vi "dectector.vi"() -> ()   [LabVIEW 2014]
uses:
  <vilib>/Analysis/2dsp.llb/1D Cross Correlation (DBL).vi
  <vilib>/Analysis/NI_AALBase.lvlib
  <vilib>/Analysis/NI_AALPro.lvlib
panel:
  out "size(s)":i32
  out "sinewave":dbl[](graph)
  out "Autocorrelacion":dynamicdata(graph)
  in  "Muestras":i32=128
  in  "Amplitud":dbl=1.0 format="%#_13g"
  in  "Ciclos":dbl
  out "Correlacion":dbl[](graph)
  out "Comparator Output":bool[](array[boolean])
  in  "Constant":i32
  out "Average Results":dbl[](array[numeric])
  out "Comparator Output":dbl[](array[numeric])
  out "Outputs":cluster{dbl, dbl}(graph)
  out "Correlation":dbl[](array[numeric])
  in  "Average Constant":i32
  in  "STOP":bool
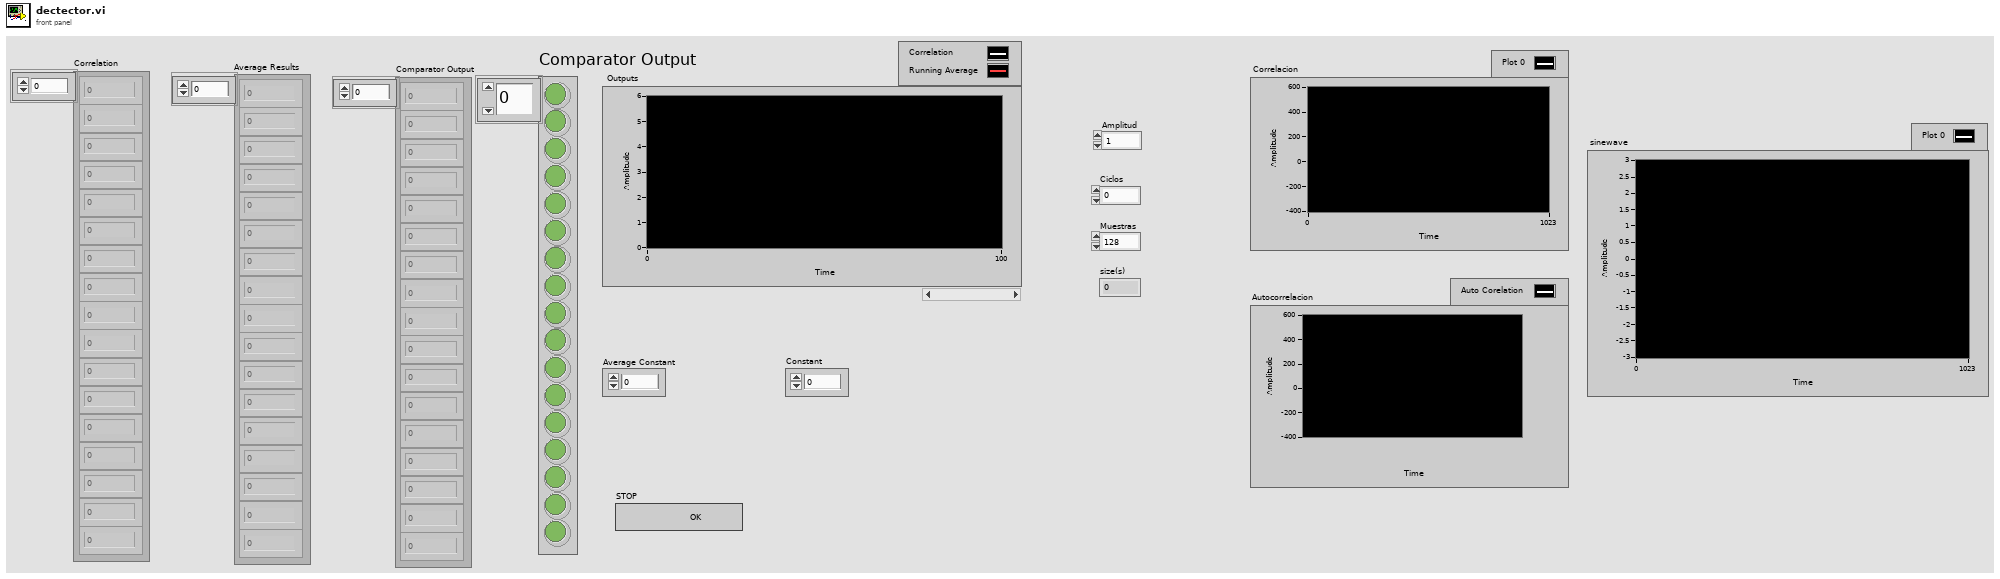
[diagram p1: front panel]
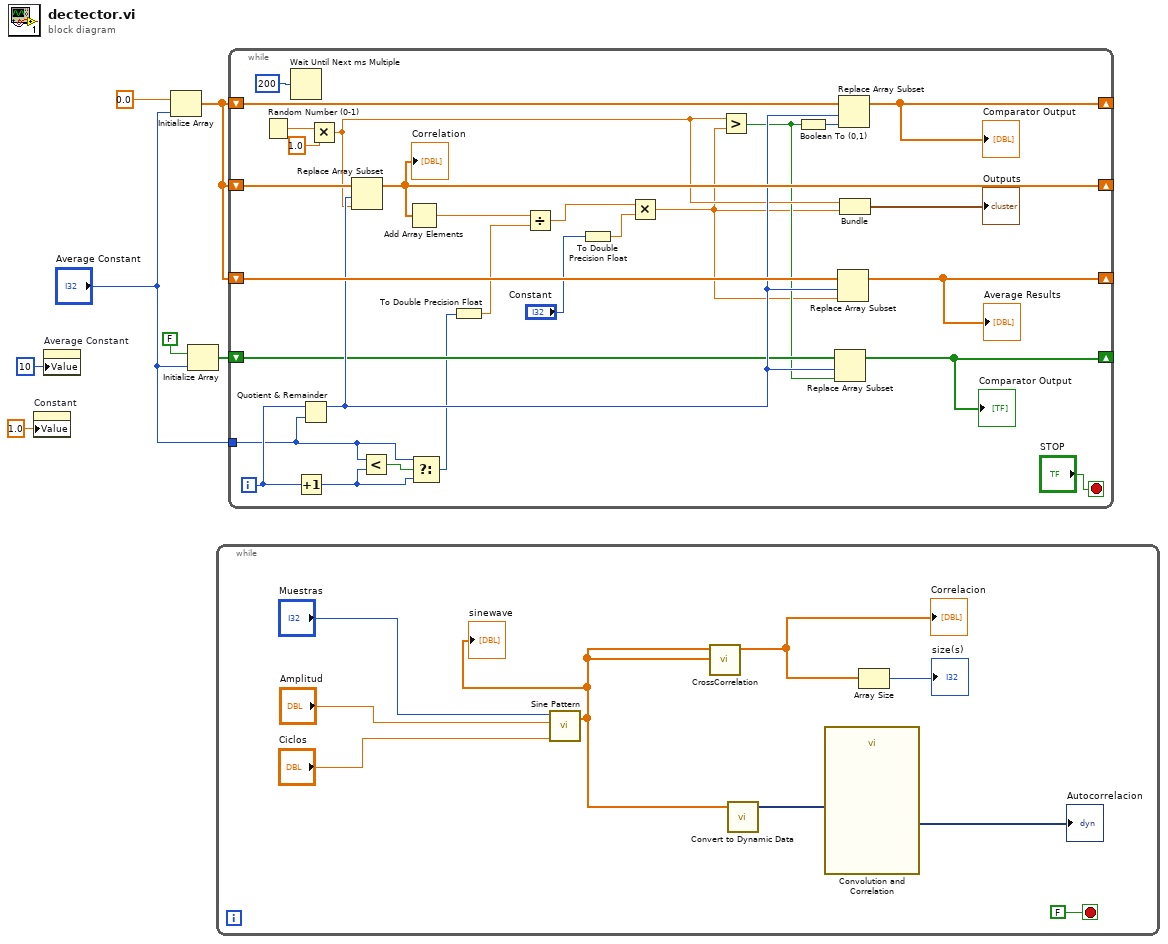
[diagram p0: block diagram]
diagram:
  n1 = property on="Constant" class="DigNum (strict)"("Value"=1.0 ("Constant")) -> ()  [unwired: 2 in, 2 out]
  n2 = property on="Average Constant" class="DigNum (strict)"("Value"=i8 10 ("Average Constant")) -> ()  [unwired: 2 in, 2 out]
  n3 = Initialize Array(0.0 ("element"), "Average Constant") -> (w6:dbl[])
  n4 = Initialize Array(FALSE, "Average Constant") -> (w3:bool[])
  n5 = while {
    stop <- FALSE stop-if-true
    n6 = call <vilib>:"Sine Pattern.vi"("cycles"="Ciclos", "amplitude"="Amplitud", "samples"="Muestras") -> ("Sinusoidal Pattern"=w10:dbl[])  [unwired: 1 in, 1 out]
    "sinewave" <- w10
    n7 = call-poly <vilib>:"CrossCorrelation.vi"("Y"=w10, "X"=w10) -> ("Rxy"=w9:dbl[])  [unwired: 8 in, 1 out]
    "Correlacion" <- w9
    n8 = call "Convert to Dynamic Data"("Array"=w10) -> ("Dynamic Data Type"=w11:dynamicdata)  [unwired: 3 in]
    n9 = call "Convolution and Correlation"("X"=w11) -> ("Rxx"=→"Autocorrelacion":dynamicdata)  [unwired: 9 in, 1 out]
    n10 = Array Size(array=w9) -> (size(s)=→"size(s)":i32)
  }
  n11 = while {
    tunnel: "Average Constant" -> [w40]
    shift-right: [w35] -> _
    shift-left: w6 -> [w37]
    shift-right: [w31] -> _
    shift-left: w6 -> [w32]
    shift-right: [w28] -> _
    shift-left: w6 -> [w29]
    shift-right: [w24] -> _
    shift-left: w3 -> [w25]
    i -> [w43]
    stop <- "STOP" stop-if-true
    n12 = Random Number (0-1)() -> (number: 0 to 1=w38:dbl)
    n13 = Wait Until Next ms Multiple(millisecond multiple=u32 200) -> ()  [unwired: 1 out]
    n14 = Increment(x=w43) -> (x+1=w41:i32)
    n15 = Quotient & Remainder(x=w43, y=w40) -> (x-y*floor(x/y)=w26:i32)  [unwired: 1 out]
    n16 = Multiply(x=w38, y=1.0) -> (x*y=w23:dbl)
    n17 = Replace Array Subset(array=w37, new element=w23, index=w26) -> (w35:dbl[])
    "Correlation" <- w35
    n18 = Less?(x=w40, y=w41) -> (x < y?=w42:bool)
    n19 = Add Array Elements(numeric array=w35) -> (sum=w36:dbl)
    n20 = Select(t=w40, s=w42, f=w41) -> (s? t:f=w20:i32)
    n21 = To Double Precision Float(number=w20) -> (double precision float=w19:dbl)
    n22 = Divide(x=w36, y=w19) -> (x/y=w27:dbl)
    n23 = To Double Precision Float(number="Constant") -> (double precision float=w17:dbl)
    n24 = Multiply(x=w27, y=w17) -> (x*y=w21:dbl)
    n25 = Greater?(x=w23, y=w21) -> (0:w22:bool)
    n26 = Boolean To (0,1)(Boolean=w22) -> (0, 1=w30:i16)
    n27 = Replace Array Subset(array=w25, new element=w22, index=w26) -> (w24:bool[])
    "Comparator Output" <- w24
    n28 = Replace Array Subset(array=w29, new element=w21, index=w26) -> (w28:dbl[])
    "Average Results" <- w28
    n29 = Replace Array Subset(array=w32, new element=w30, index=w26) -> (w31:dbl[])
    "Comparator Output" <- w31
    n30 = Bundle(w23, w21) -> (→"Outputs":cluster{dbl, dbl})  [unwired: 1 in]
  }
